vi "Read handsetOff2.vi"(8 "error in (no error)":errorcluster, 11 "OffsetStatus in":refnum<class "OffsetStatus.lvclass">) -> (0 "error out":errorcluster, 2 "handsetOff2":dbl[unit] min=-0.00048481368110953597 max=0.00048481368110953597, 3 "OffsetStatus out":refnum<class "OffsetStatus.lvclass">)   [LabVIEW 2014, in "TCSDataDefinitions.lvlib" / "TCSPublicStatus.lvlib" / "OffsetStatus.lvclass"]
uses:
  OffsetStatus.lvclass
  OffsetStatus.lvclass/OffsetStatus.ctl
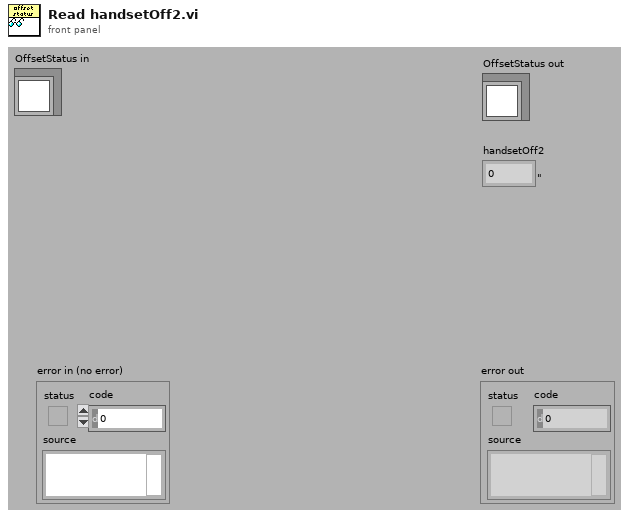
[diagram p1: front panel]
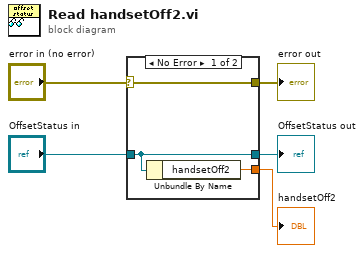
[diagram p0: block diagram]
diagram:
  n1 = case shown="No Error" "error in (no error)" {
    selector: "error in (no error)" -> [w8 w9]
    tunnel: [w8 w9] -> w4
    tunnel: [w7 w10] -> w1
    tunnel: "OffsetStatus in" -> [w7 w10]
    tunnel: [w6 _] -> w3
    frame No Error {
      n2 = Unbundle By Name(w7) -> ("handsetOff2"=w6:dbl[unit])
    }
    frame Error {
    }
  }
  "error out" <- w4
  "handsetOff2" <- w3
  "OffsetStatus out" <- w1
